vi "build_protocol.vi"(10 "Test Angles (degrees)":dbl[](array[numeric]), 11 "Trials per angle":u8) -> (1 "shuffled array":i32[](array[numeric]), 2 "Numeric":i32, 3 "Array":dbl[][](array[numeric]))   [LabVIEW 2020]
uses:
  c9ea2b35-329a-4f4d-a603-e654c0e752f1.vi
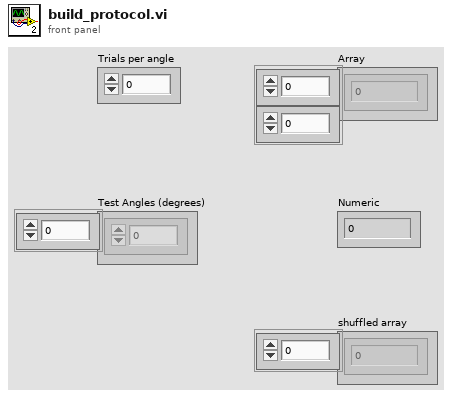
[diagram p1: front panel]
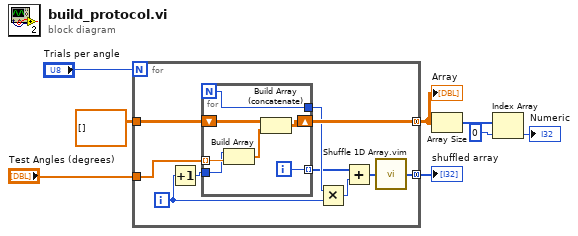
[diagram p0: block diagram]
diagram:
  n1 = for {
    N: "Trials per angle" -> [_]
    tunnel: "Test Angles (degrees)" -> [w16]
    tunnel: dbl[][] [] -> [w18]
    tunnel: [w17] -> w3 mode=concatenating
    tunnel: [w11] -> w8 mode=concatenating
    i -> [w9]
    n2 = Increment(x=w9) -> (x+1=w10:i32)
    n3 = for {
      N -> [w19]
      tunnel: w16 -> [w25] mode=indexing
      shift-right: [w22] -> w17
      shift-left: w18 -> [w23]
      tunnel: w10 -> [w21]
      tunnel: [w20] -> w14 mode=indexing
      tunnel: [w19] -> w15
      i -> [w20]
      n4 = Build Array(w21, w25) -> (w24:dbl[])
      n5 = Build Array (concatenate)(w23, w24) -> (w22:dbl[][])
    }
    n6 = Multiply(x=w15, y=w9) -> (x*y=w13:i32)
    n7 = Add(x=w14, y=w13) -> (x+y=w12:i32[])
    n8 = call "Shuffle 1D Array.vim"("array"=w12) -> ("shuffled array"=w11:i32[])  [unwired: 4 in]
  }
  "shuffled array" <- w8
  "Array" <- w3
  n9 = Array Size(array=w3) -> (size(s)=w4:i32[])
  n10 = Index Array(array=w4, index=0) -> (element=→"Numeric":i32)
